vi "EF_InsertIntoTimeTrace.vi"(6 "TimeTrace in":u32[](array[numeric]), 8 "NumVals":i32, 9 "Vals":u32[](array[numeric]), 10 "LengthTTrace":u64, 11 "TimeTraceBin":i32) -> (3 "TimeTrace out":u32[](array[numeric]))   [LabVIEW 2017]
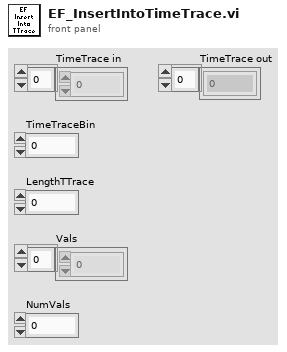
[diagram p1: front panel]
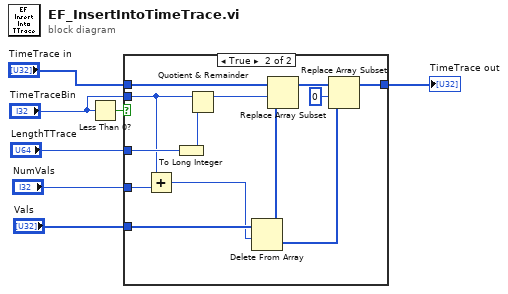
[diagram p0: block diagram]
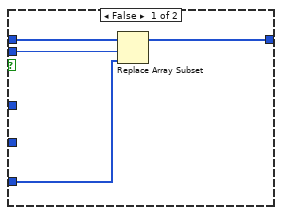
[diagram p2: hidden frame]
diagram:
  n1 = Less Than 0?(x="TimeTraceBin") -> (x < 0?=w4:bool)
  n2 = case shown="True" w4 {
    tunnel: "TimeTrace in" -> [w11 w24]
    tunnel: "Vals" -> [w10 w21]
    tunnel: [w9 w22] -> w3
    tunnel: "TimeTraceBin" -> [w8 w12]
    tunnel: "LengthTTrace" -> [_ w16]
    tunnel: "NumVals" -> [_ w13]
    frame False {
      n3 = Replace Array Subset(array=w11, new element=w10, index=w8) -> (w9:u32[])
    }
    frame True {
      n4 = Add(x=w12, y=w13) -> (x+y=w19:i32)
      n5 = To Long Integer(number=w16) -> (32bit integer=w15:i32)
      n6 = Quotient & Remainder(x=w12, y=w15) -> (x-y*floor(x/y)=w14:i32)  [unwired: 1 out]
      n7 = Delete From Array(array=w21, length=w19) -> (deleted portion=w18:u32[], array with subset deleted=w20:u32[])  [unwired: 1 in]
      n8 = Replace Array Subset(array=w24, new element=w20, index=w14) -> (w23:u32[])
      n9 = Replace Array Subset(array=w23, new element=w18, index=0) -> (w22:u32[])
    }
  }
  "TimeTrace out" <- w3
